vi "Scoring Paths.vi"(8 "error in (no error)":errorcluster, 10 "Submission":refnum<class "Submission.lvclass">, 11 "SOL-Server in":refnum<class "SOL-Server.lvclass">) -> (0 "error out":errorcluster, 3 "SOL-Server out":refnum<class "SOL-Server.lvclass">, 4 "LLB Path":path, 6 "Scorer Path":path)   [LabVIEW 2020, in "Summer of LabVIEW.lvlib" / "SOL-Server.lvclass"]
uses:
  SOL-Server.lvclass
  Submission/Submission.lvclass
  SOL-Server.lvclass/SOL-Server.ctl
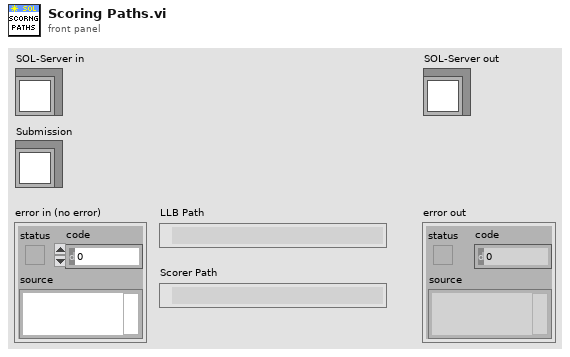
[diagram p1: front panel]
types:
  T1 = typedef "Summer of LabVIEW.lvlib/SOL-Server.lvclass/Paths.ctl" = cluster{"Web Root":path, "Sessions":path, "Config":path, "SQLite DB File":path, "SSL Cert Folder":path, "Submissions":path, "Scorers":path}
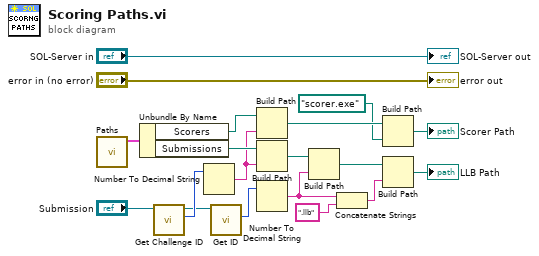
[diagram p0: block diagram]
diagram:
  n1 = call "Paths.vi"() -> ("Paths"=w17:T1)  [unwired: 11 in]
  n2 = Unbundle By Name(w17) -> ("Scorers"=w8:path, "Submissions"=w14:path)
  n3 = call "Get Challenge ID.vi"("Submission in"="Submission") -> ("Challenge ID"=w15:i64, "Submission out"=w2:refnum<class "Submission.lvclass">)  [unwired: 9 in]
  n4 = Number To Decimal String(number=w15) -> (decimal integer string=w3:string)  [unwired: 1 in]
  n5 = call "Get ID.vi"("Submission in"=w2) -> ("ID"=w16:i64)  [unwired: 9 in, 1 out]
  n6 = Build Path(base path=w8, name or relative path=w3) -> (appended path=w7:path)
  n7 = Build Path(base path=w14, name or relative path=w3) -> (appended path=w13:path)
  n8 = Number To Decimal String(number=w16) -> (decimal integer string=w4:string)  [unwired: 1 in]
  n9 = Build Path(base path=w13, name or relative path=w4) -> (appended path=w11:path)
  n10 = Concatenate Strings(w4, ".llb" ("string")) -> (w10:string)
  n11 = Build Path(base path=w7, name or relative path=path "scorer.exe") -> (appended path=→"Scorer Path":path)
  n12 = Build Path(base path=w11, name or relative path=w10) -> (appended path=→"LLB Path":path)
  "error out" <- "error in (no error)"
  "SOL-Server out" <- "SOL-Server in"
